vi "is valid.vi"(11 "connection in":refnum<class "connection maintainer.lvclass">) -> (3 "valid":bool)   [LabVIEW 2015, in "connection maintainer.lvclass"]
uses:
  connection maintainer.lvclass
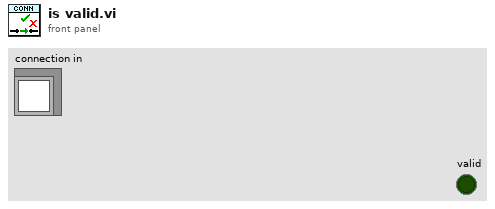
[diagram p1: front panel]
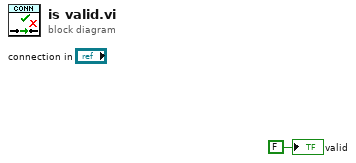
[diagram p0: block diagram]
diagram:
  "valid" <- FALSE ("valid")
